vi "ParseDataa.vi"(9 "data out":string) -> (0 "Sensor data 4":T1, 1 "Sensor data 3":T1, 2 "Sensor data 2":T1, 3 "Sensor data 1":T1, 4 "Sensor data 6":T1, 5 "Sensor data 5":T1, 6 "BSN":u8, 7 "lock":u8, 11 "GTS Fields":T2)   [LabVIEW 2011]
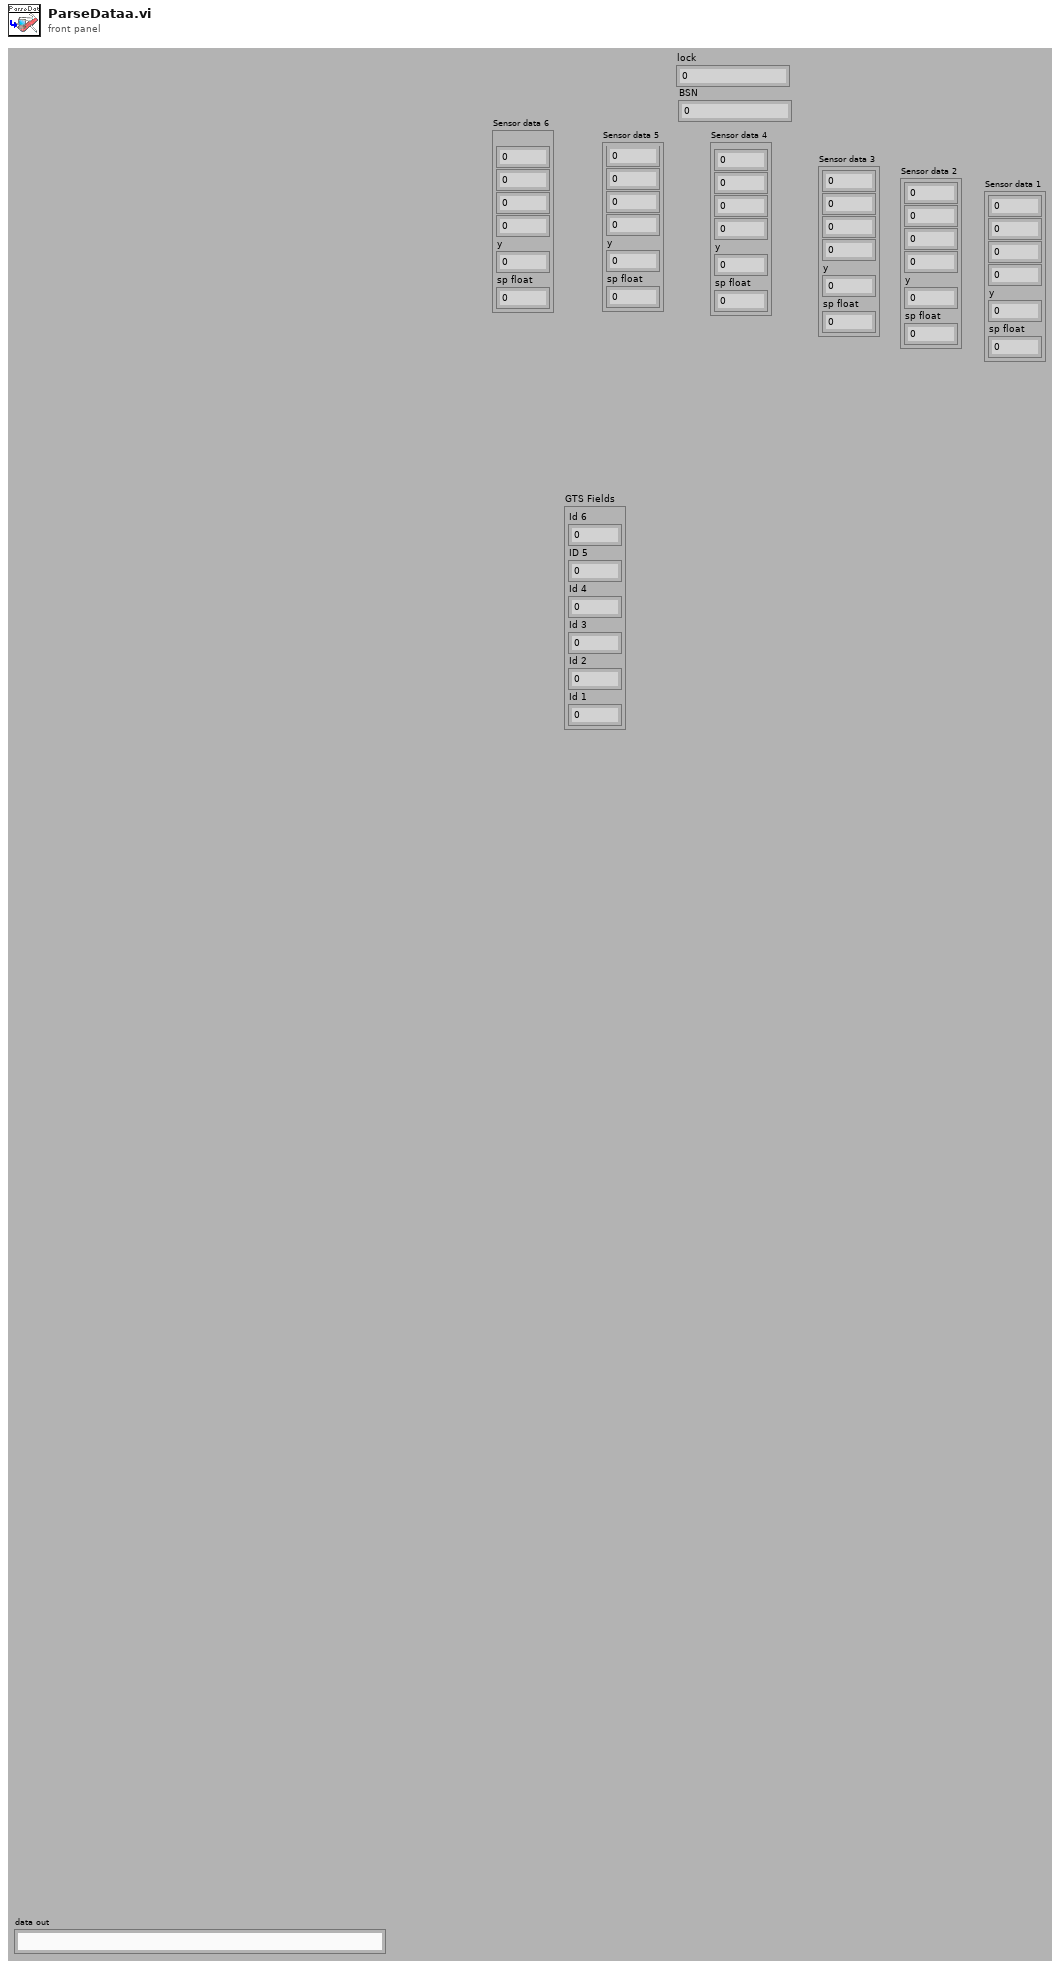
[diagram p1: front panel]
types:
  T1 = cluster{dbl, dbl, dbl, dbl, "y":dbl, "sp float":u8}
  T2 = cluster{"Id 6":u8, "ID 5":u8, "Id 4":u8, "Id 3":u8, "Id 2":u8, "Id 1":u8}
  T3 = cluster{"sp float":u8, "sp float":u8, "sp float":u8, "sp float":u8, "sp float":u8, "sp float":u8}
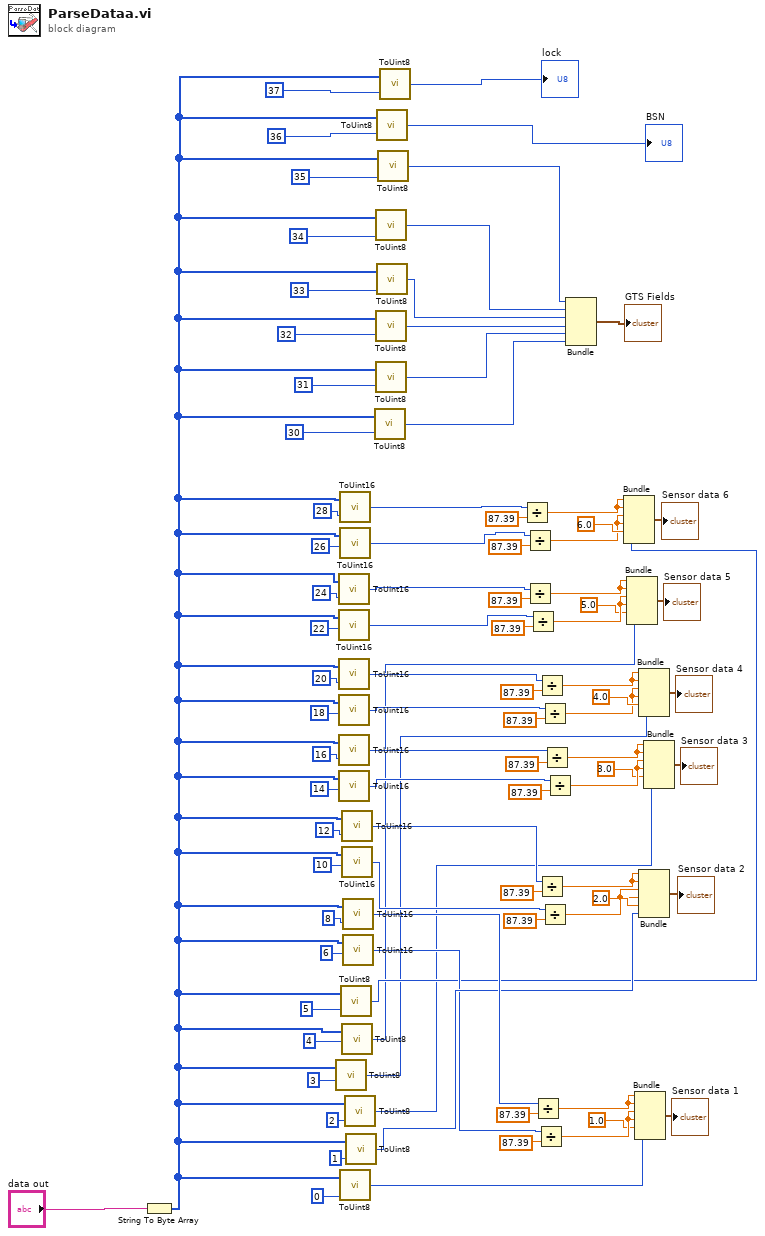
[diagram p0: block diagram]
diagram:
  n1 = String To Byte Array(string="data out") -> (unsigned byte array=w5:u8[])
  n2 = call "ToUint8.vi"("index"=3, "array"=w5) -> ("sp float"=w7:u8)
  n3 = call "ToUint16.vi"("index"=24, "array"=w5) -> ("sp float"=w18:u16)
  n4 = call "ToUint16.vi"("index"=22, "array"=w5) -> ("sp float"=w19:u16)
  n5 = call "ToUint16.vi"("index"=20, "array"=w5) -> ("sp float"=w21:u16)
  n6 = call "ToUint16.vi"("index"=18, "array"=w5) -> ("sp float"=w20:u16)
  n7 = call "ToUint16.vi"("index"=16, "array"=w5) -> ("sp float"=w23:u16)
  n8 = call "ToUint16.vi"("index"=14, "array"=w5) -> ("sp float"=w22:u16)
  n9 = call "ToUint16.vi"("index"=28, "array"=w5) -> ("sp float"=w11:u16)
  n10 = call "ToUint16.vi"("index"=26, "array"=w5) -> ("sp float"=w10:u16)
  n11 = call "ToUint8.vi"("index"=0, "array"=w5) -> ("sp float"=w54:u8)
  n12 = call "ToUint8.vi"("index"=5, "array"=w5) -> ("sp float"=w9:u8)
  n13 = call "ToUint16.vi"("index"=12, "array"=w5) -> ("sp float"=w45:u16)
  n14 = call "ToUint16.vi"("index"=10, "array"=w5) -> ("sp float"=w44:u16)
  n15 = call "ToUint8.vi"("index"=4, "array"=w5) -> ("sp float"=w8:u8)
  n16 = call "ToUint16.vi"("index"=8, "array"=w5) -> ("sp float"=w58:u16)
  n17 = call "ToUint16.vi"("index"=6, "array"=w5) -> ("sp float"=w42:u16)
  n18 = call "ToUint8.vi"("index"=2, "array"=w5) -> ("sp float"=w6:u8)
  n19 = call "ToUint8.vi"("index"=1, "array"=w5) -> ("sp float"=w43:u8)
  n20 = call "ToUint8.vi"("index"=30, "array"=w5) -> ("sp float"=w65:u8)
  n21 = call "ToUint8.vi"("index"=34, "array"=w5) -> ("sp float"=w69:u8)
  n22 = call "ToUint8.vi"("index"=32, "array"=w5) -> ("sp float"=w67:u8)
  n23 = call "ToUint8.vi"("index"=31, "array"=w5) -> ("sp float"=w66:u8)
  n24 = call "ToUint8.vi"("index"=36, "array"=w5) -> ("sp float"=→"BSN":u8)
  n25 = call "ToUint8.vi"("index"=33, "array"=w5) -> ("sp float"=w68:u8)
  n26 = call "ToUint8.vi"("index"=35, "array"=w5) -> ("sp float"=w70:u8)
  n27 = call "ToUint8.vi"("index"=37, "array"=w5) -> ("sp float"=→"lock":u8)
  n28 = Divide(x=w11, y=87.39) -> (x/y=w13:dbl)
  n29 = Divide(x=w10, y=87.39) -> (x/y=w15:dbl)
  n30 = Divide(x=w18, y=87.39) -> (x/y=w28:dbl)
  n31 = Divide(x=w19, y=87.39) -> (x/y=w26:dbl)
  n32 = Divide(x=w58, y=87.39) -> (x/y=w57:dbl)
  n33 = Divide(x=w42, y=87.39) -> (x/y=w55:dbl)
  n34 = Divide(x=w21, y=87.39) -> (x/y=w31:dbl)
  n35 = Divide(x=w45, y=87.39) -> (x/y=w47:dbl)
  n36 = Divide(x=w20, y=87.39) -> (x/y=w33:dbl)
  n37 = Divide(x=w44, y=87.39) -> (x/y=w49:dbl)
  n38 = Divide(x=w23, y=87.39) -> (x/y=w40:dbl)
  n39 = Divide(x=w22, y=87.39) -> (x/y=w38:dbl)
  n40 = Bundle("sp float"=w70, "sp float"=w69, "sp float"=w68, "sp float"=w67, "sp float"=w66, "sp float"=w65) -> (→"GTS Fields":T3)  [unwired: 1 in]
  n41 = Bundle(w13, w13, w15, w15, "y"=6.0, "sp float"=w9) -> (→"Sensor data 6":T1)  [unwired: 1 in]
  n42 = Bundle(w28, w28, w26, w26, "y"=5.0, "sp float"=w8) -> (→"Sensor data 5":T1)  [unwired: 1 in]
  n43 = Bundle(w57, w57, w55, w55, "y"=1.0, "sp float"=w54) -> (→"Sensor data 1":T1)  [unwired: 1 in]
  n44 = Bundle(w31, w31, w33, w33, "y"=4.0, "sp float"=w7) -> (→"Sensor data 4":T1)  [unwired: 1 in]
  n45 = Bundle(w47, w47, w49, w49, "y"=2.0, "sp float"=w43) -> (→"Sensor data 2":T1)  [unwired: 1 in]
  n46 = Bundle(w40, w40, w38, w38, "y"=3.0, "sp float"=w6) -> (→"Sensor data 3":T1)  [unwired: 1 in]
